vi "Setup.vi"(8 "error in":errorcluster, 11 "VISA resource name":refnum<visa-resource-name>) -> (0 "error out":errorcluster, 3 "Megger cluster out":T1={"Read data"={"Firmware version"="", "Model number"="", "Serial number"=0, "Ramp rate"=0.0, "Test Voltage"=0.0, "Test duration"=0.0, "Test stop watch"=0.0, "measured Current (nA)"=0.0, "calculated Resistance"=0.0, "Test Mode"=enum."Insulation resistance (IR)", "Test status"=enum."Waiting to start test"}, "Connected?"=FALSE, "Device status array"=[]})   [LabVIEW 2014]
doc: "This function firstly configures the Serial port and then writes a list of commands to initialise the device. This function will return device information data. NOTE: This VI will take 25 seconds to capture data from device and will be locked out during this period. If an error occurs it stops immediately."
uses:
  Private/Controls/Megger cluster.ctl
  <vilib>/Instr/_visa.llb/VISA Set IO Buffer Mask.ctl
  <vilib>/Instr/_visa.llb/VISA Configure Serial Port (Instr).vi
  Private/Controls/Global Megger.vi
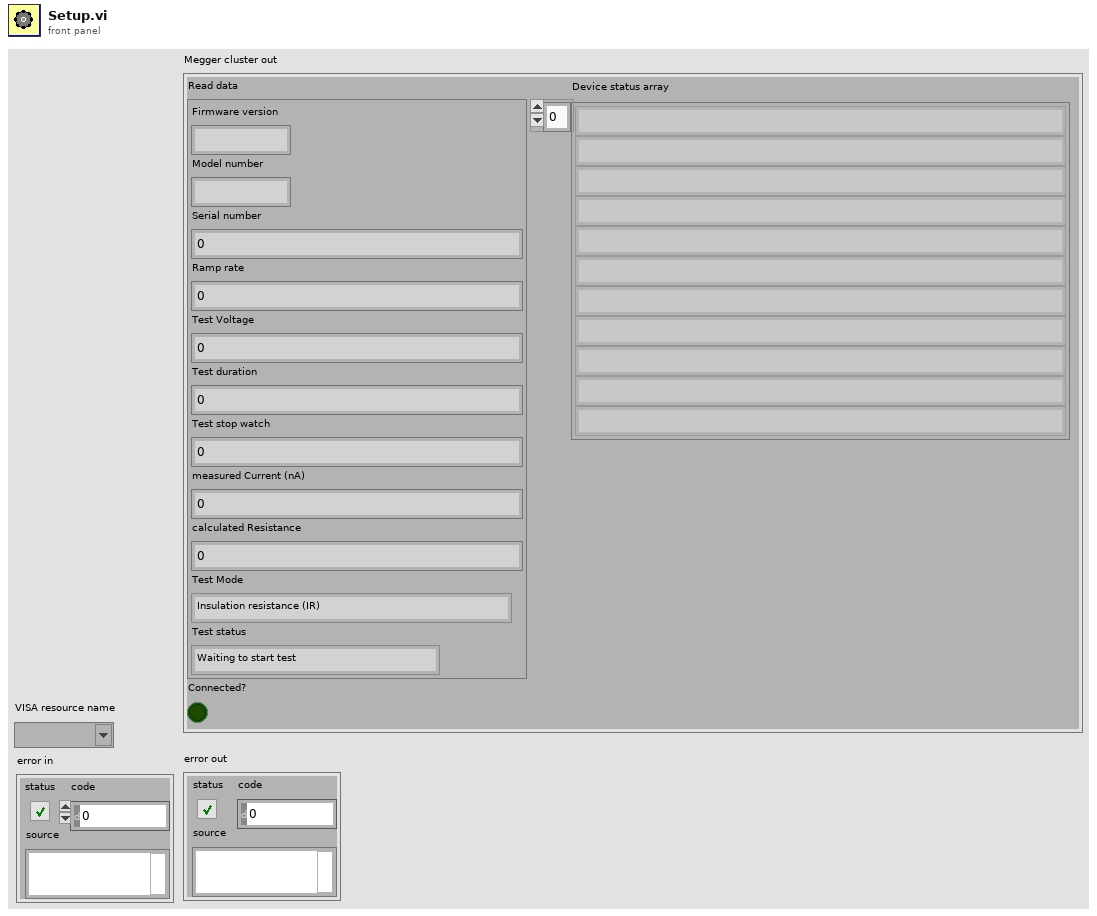
[diagram p1: front panel]
types:
  T1 = typedef "Megger cluster.ctl" = cluster{"Read data":cluster{"Firmware version":string, "Model number":string, "Serial number":i32, "Ramp rate":dbl, "Test Voltage":dbl, "Test duration":sgl, "Test stop watch":sgl, "measured Current (nA)":dbl, "calculated Resistance":dbl, "Test Mode":enum16{"N/A", "Insulation resistance (IR)", "Timed Insulation resistance (IR(t))", "Diaelectric Absorption Ratio (DAR)", "Polarisation Index (PI)", "Diaelectric Dishcharge (DD)", "Step voltage (SV)", "Ramp test (Ramp)"}, "Test status":enum16{"Waiting to start test", "Unable to start test", "Test progressing normally", "Performing post test measurements", "Test has ended normally", "Test has been aborted"}}, "Connected?":bool, "Device status array":string[]}
  T2 = typedef "VISA Set IO Buffer Mask.ctl" = u16
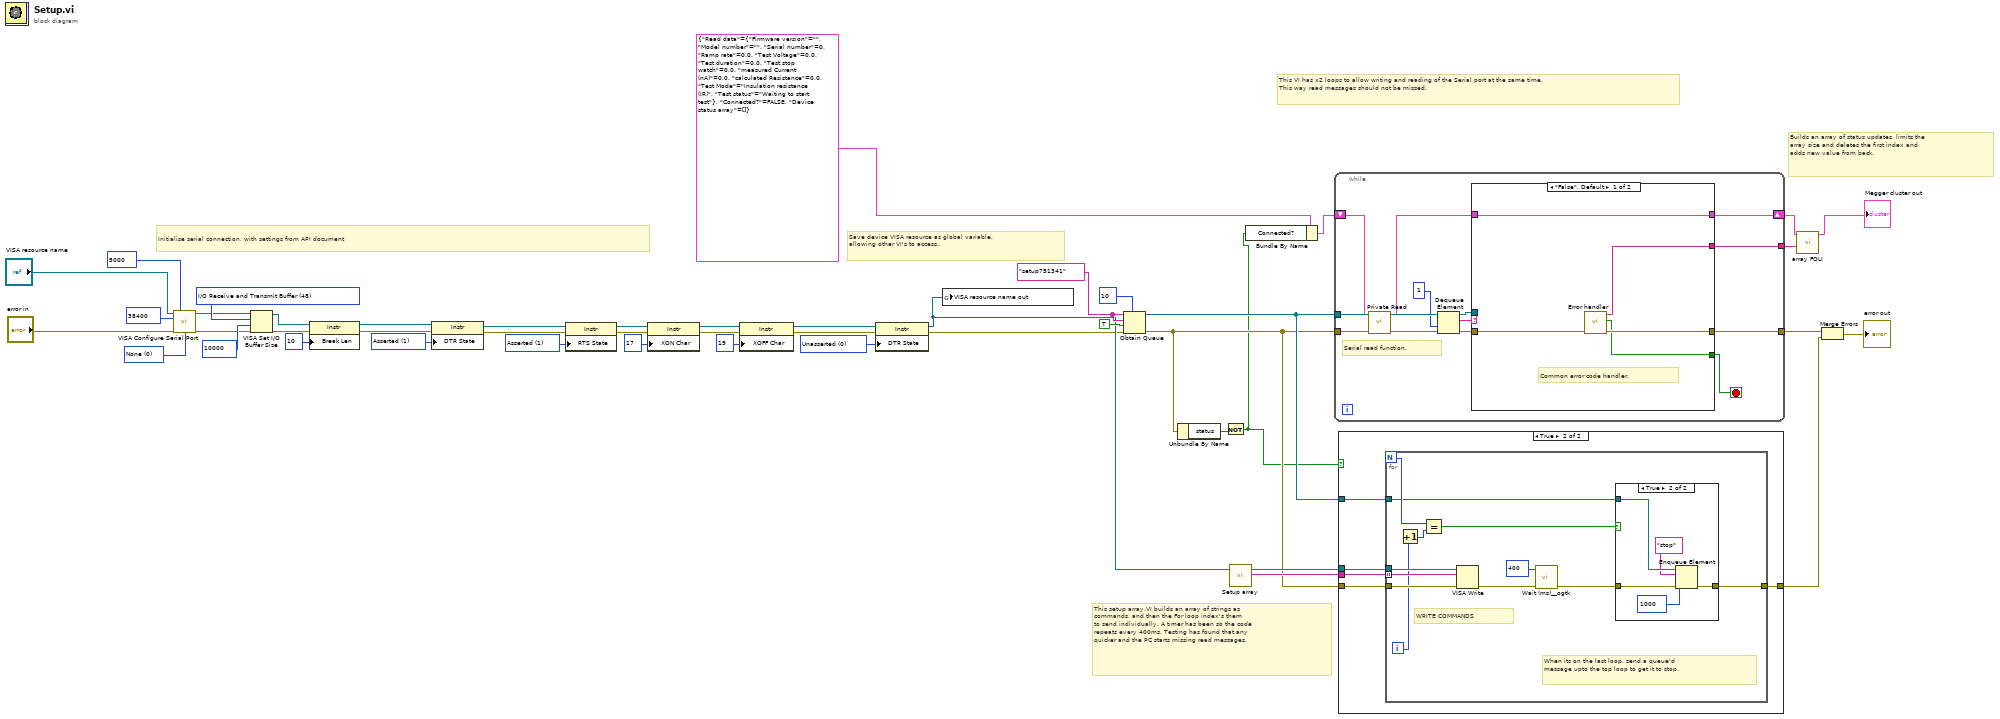
[diagram p0: block diagram]
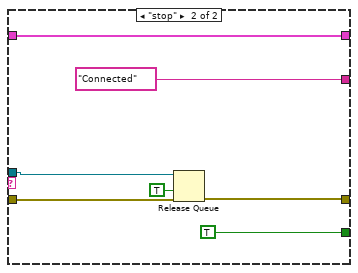
[diagram p2: hidden frame]
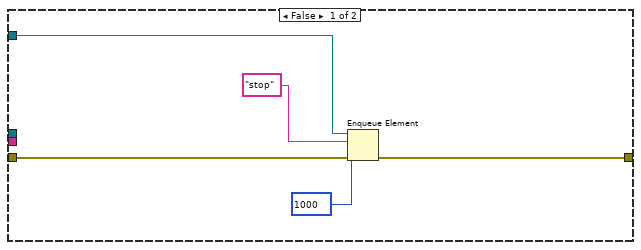
[diagram p3: hidden frame]
diagram:
  w8 = i16 0 items=["Unknown"=-1, "Unasserted"=0, "Asserted"=1] ("Serial Settings:Modem Line Settings:Line DTR State")
  w17 = i16 1 items=["Unknown"=-1, "Unasserted"=0, "Asserted"=1] ("Serial Settings:Modem Line Settings:Line RTS State")
  w18 = i16 1 items=["Unknown"=-1, "Unasserted"=0, "Asserted"=1] ("Serial Settings:Modem Line Settings:Line DTR State")
  w32 = "setup751341" ("name (unnamed)")
  w41 = u16 0 items=["None", "XON/XOFF", "RTS/CTS", "XON/XOFF & RTS/CTS", "DTR/DSR", "XON/XOFF & DTR/DSR"] ("flow control (0:none)")
  w45 = T2 48 items=["I/O Receive Buffer"=16, "I/O Transmit Buffer"=32, "I/O Receive and Transmit Buffer"=48] ("Mask")
  # "Builds an array of status updates, limits the\narray size and deletes the first index and \nadds new value from back."
  # "This setup array.VI builds an array of strings as\ncommands, and then the For loop index's them\nto send individually. A timer has been so the code\nrepeats every 400ms. Testing has found that any\nquicker and the PC starts missing read messages."
  # "This VI has x2 loops to allow writing and reading of the Serial port at the same time. \nThis way read messages should not be missed."
  # "Save device VISA resource as global variable,\nallowing other VI's to access.,"
  # "Initialise serial connection, with settings from API document"
  n1 = call-poly "VISA Configure Serial Port"("VISA resource name"="VISA resource name", "timeout (10sec)"=u32 5000, "baud rate (9600)"=u32 38400, "error in (no error)"="error in", "flow control (0:none)"=w41) -> ("VISA resource name out"=w35:refnum<visa-resource-name>, "error out"=w36:errorcluster)  [unwired: 9 in]
  n2 = VISA Set I/O Buffer Size(VISA resource name=w35, mask (16)=w45, size (4096)=u32 10000, error in (no error)=w36) -> (VISA resource name out=w42:refnum<visa-resource-name>, error out=w43:errorcluster)
  n3 = property class="Instr"(reference=w42, error in=w43, "Break Len"=i16 10 ("Serial Settings:Break Length")) -> (reference out=w10:refnum<visa-resource-name>, error out=w11:errorcluster)
  n4 = property class="Instr"(reference=w10, error in=w11, "DTR State"=w18) -> (reference out=w16:refnum<visa-resource-name>, error out=w23:errorcluster)
  n5 = property class="Instr"(reference=w16, error in=w23, "RTS State"=w17) -> (reference out=w15:refnum<visa-resource-name>, error out=w22:errorcluster)
  n6 = property class="Instr"(reference=w15, error in=w22, "XON Char"=u8 17 ("Serial Settings:Flow Control XON Character")) -> (reference out=w14:refnum<visa-resource-name>, error out=w21:errorcluster)
  n7 = property class="Instr"(reference=w14, error in=w21, "XOFF Char"=u8 19 ("Serial Settings:Flow Control XOFF Character")) -> (reference out=w13:refnum<visa-resource-name>, error out=w12:errorcluster)
  n8 = property class="Instr"(reference=w13, error in=w12, "DTR State"=w8) -> (reference out=w28:refnum<visa-resource-name>, error out=w27:errorcluster)
  n9 = global write "Global Megger.vi" "VISA resource name out"(w28) -> ()
  n10 = Obtain Queue(max queue size (-1, unlimited)=10, name (unnamed)=w32, element data type=w32, create if not found? (T)=TRUE, error in (no error)=w27) -> (queue out=w30:refnum<queue>, error out=w25:errorcluster)  [unwired: 1 out]
  n11 = Unbundle By Name(w25) -> ("status"=w24:bool)
  n12 = Not(x=w24) -> (.not. x?=w5:bool)
  n13 = call "Setup array.vi"() -> ("output array"=w26:string[])  [unwired: 11 in]
  n14 = Bundle By Name(cluster=T1 {"Read data"={"Firmware version"="", "Model number"="", "Serial number"=0, "Ramp rate"=0.0, "Test Voltage"=0.0, "Test duration"=0.0, "Test stop watch"=0.0, "measured Current (nA)"=0.0, "calculated Resistance"=0.0, "Test Mode"=enum."Insulation resistance (IR)", "Test status"=enum."Waiting to start test"}, "Connected?"=FALSE, "Device status array"=[]} ("Read data"), "Connected?"=w5) -> (w6:T1)
  n15 = while {
    tunnel: w25 -> [w54]
    tunnel: w30 -> [w58]
    tunnel: [w50] -> w29
    shift-right: [w47] -> w3
    shift-left: w6 -> [w53]
    tunnel: [w46] -> w4
    stop <- w51 stop-if-true
    # "Serial read function."
    n16 = call "Private Read.vi"("error in"=w54, "Megger cluster in"=w53) -> ("error out"=w55:errorcluster, "Megger cluster out"=w52:T1)  [unwired: 7 in, 1 out]
    n17 = Dequeue Element(queue=w58, timeout in ms (-1)=1, error in (no error)=w55) -> (queue out=w48:refnum<queue>, element=w57:string, error out=w49:errorcluster)  [unwired: 1 out]
    n18 = case shown="\"False\", Default" w57 {
      tunnel: w52 -> [w63 w69]
      tunnel: [w59 TRUE] -> w51
      tunnel: [w63 w69] -> w47
      tunnel: [w60 w67] -> w50
      tunnel: w49 -> [w62 w68]
      tunnel: w48 -> [_ w66]
      tunnel: [w61 "Connected"] -> w46
      frame "False", Default {
        # "Common error code handler."
        n19 = call "Error handler.vi"("error in"=w62) -> ("error out"=w60:errorcluster, "status"=w59:bool, "Status string"=w61:string)  [unwired: 8 in]
      }
      frame "stop" {
        n20 = Release Queue(queue=w66, force destroy? (F)=TRUE, error in (no error)=w68) -> (error out=w67:errorcluster)  [unwired: 2 out]
      }
    }
  }
  n21 = case shown="True" w5 {
    tunnel: w26 -> [_ w80]
    tunnel: w25 -> [w72 w79]
    tunnel: w28 -> [_ w78]
    tunnel: [w71 w77] -> w34
    tunnel: w30 -> [w73 w76]
    frame False {
      n22 = Enqueue Element(queue=w73, element="stop", timeout in ms (-1)=1000, error in (no error)=w72) -> (error out=w71:errorcluster)  [unwired: 2 out]
    }
    frame True {
      n23 = for {
        N -> [w87]
        tunnel: w80 -> [w92] mode=indexing
        tunnel: w79 -> [w91]
        tunnel: w78 -> [w90]
        tunnel: [w83] -> w77
        tunnel: w76 -> [w85]
        i -> [w82]
        # "When its on the last loop, send a queue'd\nmessage upto the top loop to get it to stop."
        # "WRITE COMMANDS"
        n24 = Increment(x=w82) -> (x+1=w81:i32)
        n25 = Equal?(x=w87, y=w81) -> (x = y?=w86:bool)
        n26 = VISA Write(VISA resource name=w90, write buffer=w92, error in (no error)=w91) -> (error out=w89:errorcluster)  [unwired: 2 out]
        n27 = call <userlib>:"Wait (ms)__ogtk.vi"("error in (no error)"=w89, "milliseconds to wait"=u32 400) -> ("error out"=w84:errorcluster)  [unwired: 8 in, 1 out]
        n28 = case shown="True" w86 {
          tunnel: w85 -> [_ w98]
          tunnel: w84 -> [w93 w97]
          tunnel: [w93 w96] -> w83
          frame False {
          }
          frame True {
            n29 = Enqueue Element(queue=w98, element="stop", timeout in ms (-1)=1000, error in (no error)=w97) -> (error out=w96:errorcluster)  [unwired: 2 out]
          }
        }
      }
    }
  }
  n30 = call "array FOLI.vi"("status string"=w4, "Megger cluster in"=w3) -> ("Megger cluster out"=→"Megger cluster out":T1)  [unwired: 9 in]
  n31 = Merge Errors(w29, w34) -> (→"error out":errorcluster)
